vi "Destroy Connection Factory.vi"(8 "error in (no error)":errorcluster, 11 "IConnectionFactory in":refnum<class "IConnectionFactory.lvclass">) -> (0 "error out":errorcluster)   [LabVIEW 2019, in "IConnectionFactory.lvclass"]
uses:
  <vilib>/gpm_packages/@cs/Network-interface/Source/IConnectionFactory/IConnectionFactory.lvclass
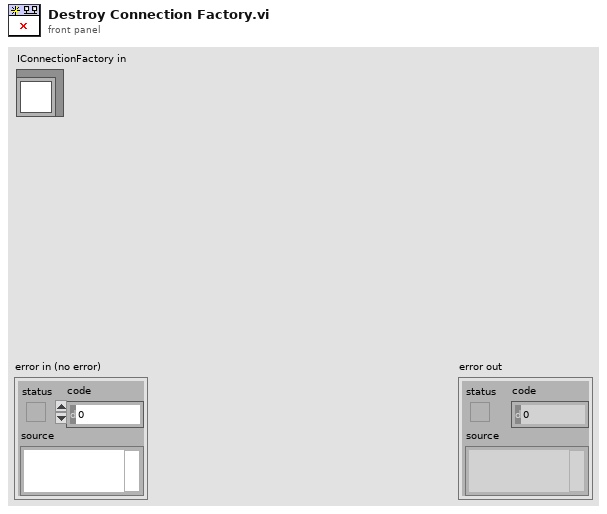
[diagram p1: front panel]
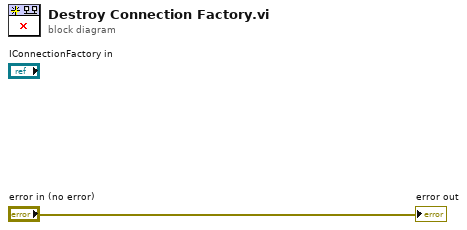
[diagram p0: block diagram]
diagram:
  "error out" <- "error in (no error)"
